vi "initialize averaging variables.vi"(4 "# of  power factor reads to avg":i32, 8 "error in (no error)":errorcluster, 10 "# of ESR reads to  average":i32, 11 "Processing loop variables":T1 {"CurrInverter"."last updated" format="%<%H:%M\n%d/%m/%Y>T"; "CurrInverter"."set flag" items=["False", "True"]}) -> (0 "error out":errorcluster, 3 "Processing loop variables out":T1 {"CurrInverter"."last updated" format="%<%H:%M\n%d/%m/%Y>T"; "CurrInverter"."set flag" items=["False", "True"]})   [LabVIEW 2019, in "Main.lvclass"]
doc: "Developed by Kevin Thompson\nkevin@thompsonengineering.net\n\nCopyright 2020\nThompson Engineering, LLC"
uses:
  Main.lvclass
  DataTypes/Processing loop variables--cluster.ctl
  DataTypes/averaging variables.ctl
  DataTypes/ESR alarm variables.ctl
  Common/DataTypes/Inverter database record v2--cluster.ctl
  Common/DataTypes/inverter info v2--cluster.ctl
  Common/DataTypes/inverter gain range--cluster.ctl
  Common/DataTypes/inverter offset range--cluster.ctl
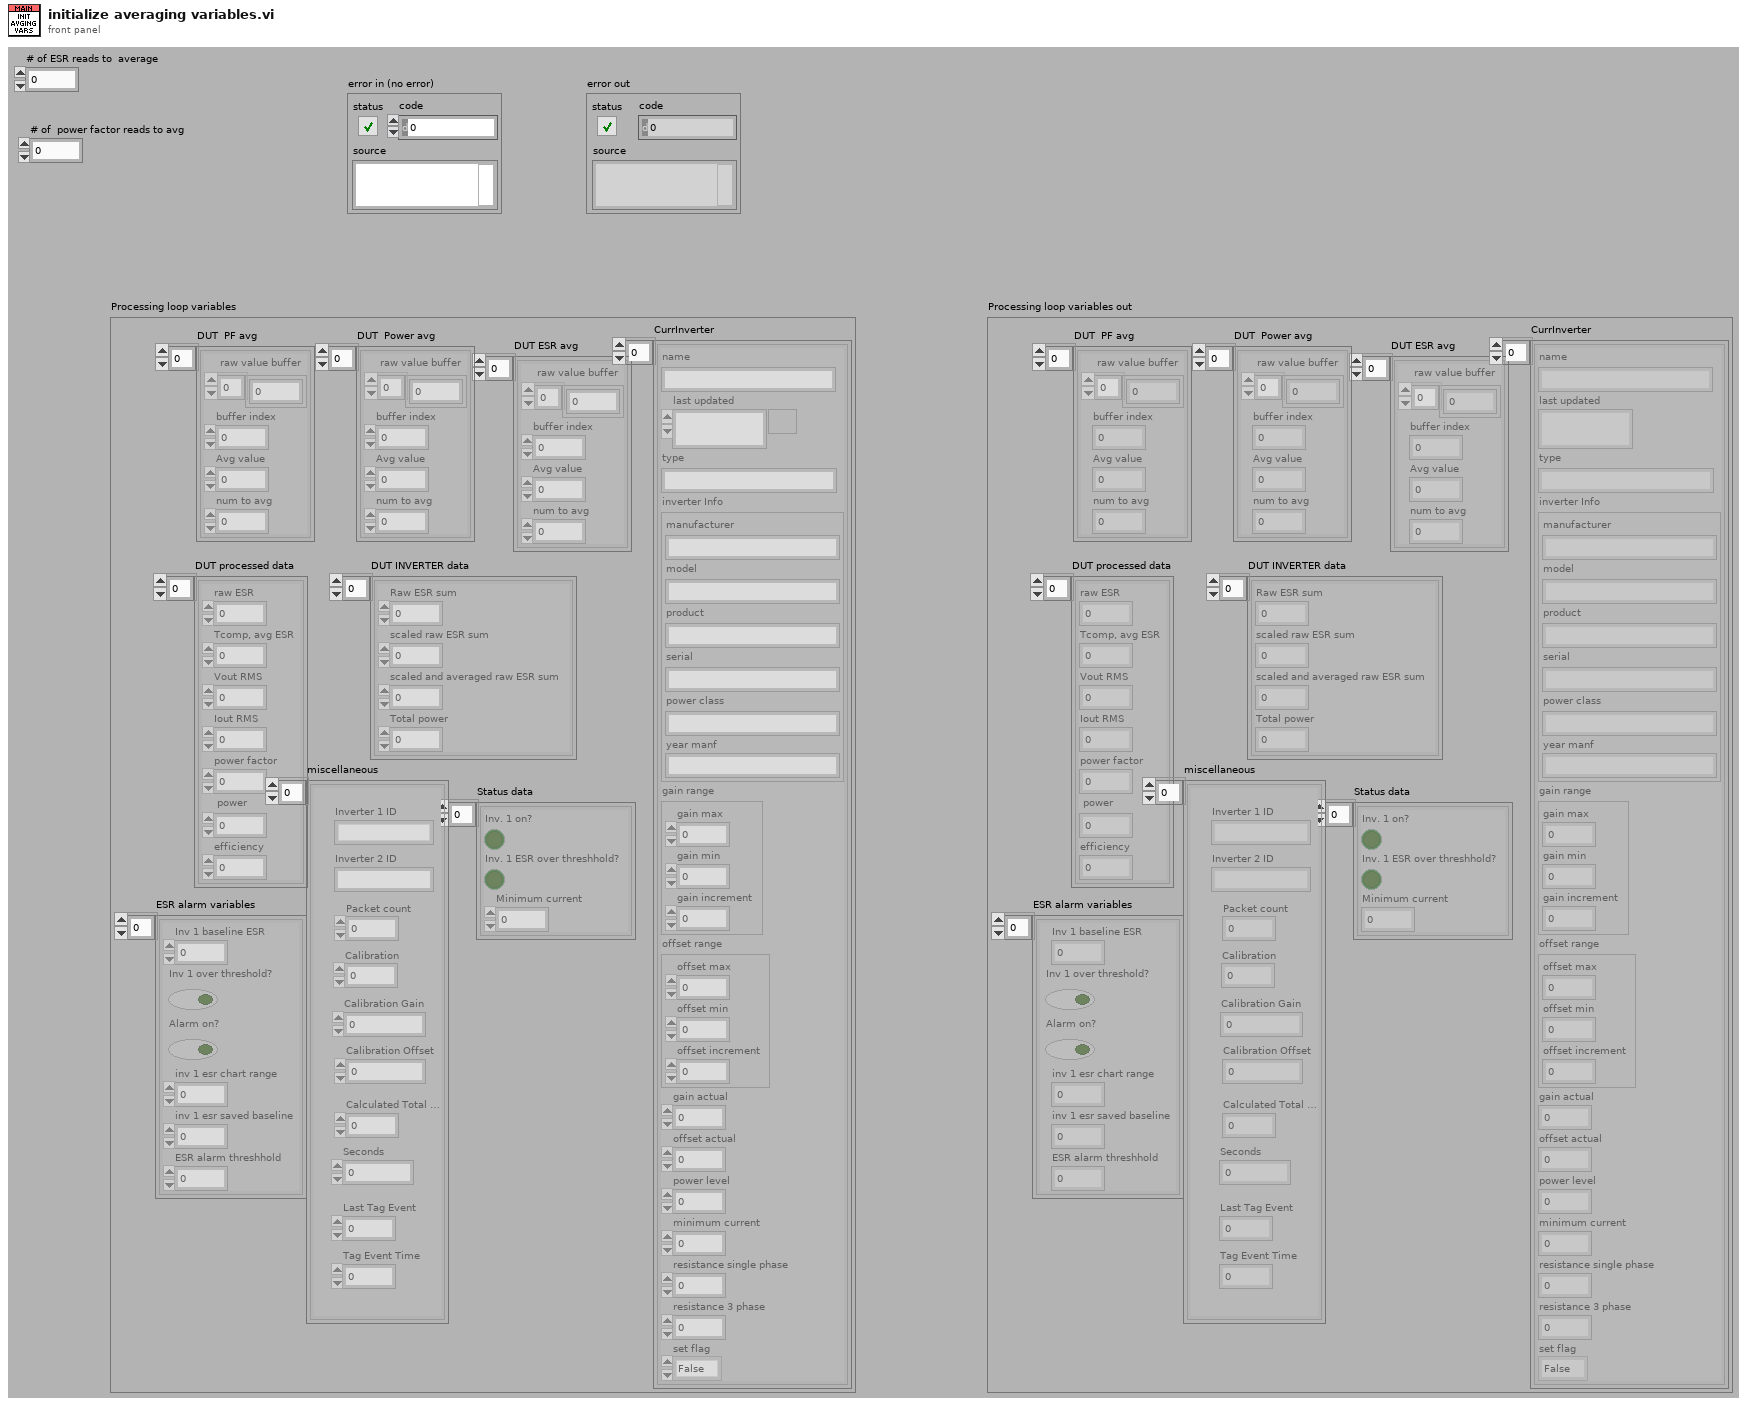
[diagram p1: front panel]
types:
  T1 = typedef "Main.lvclass/Processing loop variables--cluster.ctl" = cluster{"DUT ESR avg":T2[], "DUT  PF avg":T2[], "DUT  Power avg ":T2[], "DUT processed data":cluster{"raw ESR":dbl, "Tcomp, avg ESR":dbl, "Vout RMS":dbl, "Iout RMS":dbl, "power factor":dbl, "power":dbl, "efficiency":dbl}[], "ESR alarm variables":T3[], "Status data":cluster{"Inv. 1 on?":bool, "Inv. 1 ESR over threshhold?":bool, "Minimum current":dbl}[], "CurrInverter":T4[], "miscellaneous":cluster{"Inverter 1 ID":string, "Inverter 2 ID":string, "Packet count":u32, "Calibration":dbl, "Calibration Gain":dbl, "Calibration Offset":dbl, "Calculated Total Power":dbl, "Seconds":dbl, "Last Tag Event":dbl, "Tag Event Time":dbl}[], "DUT INVERTER data":cluster{"Raw ESR sum":dbl, "scaled raw ESR sum":dbl, "scaled and averaged raw ESR sum":dbl, "Total power":dbl}[]}
  T2 = typedef "Main.lvclass/averaging variables.ctl" = cluster{"raw value buffer":dbl[], "buffer index":i32, "Avg value":dbl, "num to avg":i32}
  T3 = typedef "Main.lvclass/ESR alarm variables.ctl" = cluster{"Inv 1 baseline ESR":dbl, "Inv 1 over threshold?":bool, "Alarm on?":bool, "inv 1 esr chart range":dbl, "inv 1 esr saved baseline":dbl, "ESR alarm threshhold":dbl}
  T4 = typedef "Inverter database record v2--cluster.ctl" = cluster{"name":string, "last updated":timestamp, "type":string, "inverter Info":T5, "gain range":T6, "offset range":T7, "gain actual":dbl, "offset actual":dbl, "power level":dbl, "minimum current":dbl, "resistance single phase":dbl, "resistance 3 phase":dbl, "set flag":u16}
  T5 = typedef "inverter info v2--cluster.ctl" = cluster{"manufacturer":string, "model":string, "product":string, "serial":string, "power class":string, "year manf":string}
  T6 = typedef "inverter gain range--cluster.ctl" = cluster{"gain max":dbl, "gain min":dbl, "gain increment":dbl}
  T7 = typedef "inverter offset range--cluster.ctl" = cluster{"offset max":dbl, "offset min":dbl, "offset increment":dbl}
  T8 = cluster{"Raw ESR sum":dbl, "scaled raw ESR sum":dbl, "scaled and averaged raw ESR sum":dbl, "Total power":dbl}
  T9 = cluster{"raw ESR":dbl, "Tcomp, avg ESR":dbl, "Vout RMS":dbl, "Iout RMS":dbl, "power factor":dbl, "power":dbl, "efficiency":dbl}
  T10 = cluster{"raw ESR":dbl, "Tcomp, avg ESR":dbl, "Vout RMS":dbl, "Iout RMS":dbl, "power factor":dbl, "power":dbl, "efficiency":dbl}[]
  T11 = cluster{"Raw ESR sum":dbl, "scaled raw ESR sum":dbl, "scaled and averaged raw ESR sum":dbl, "Total power":dbl}[]
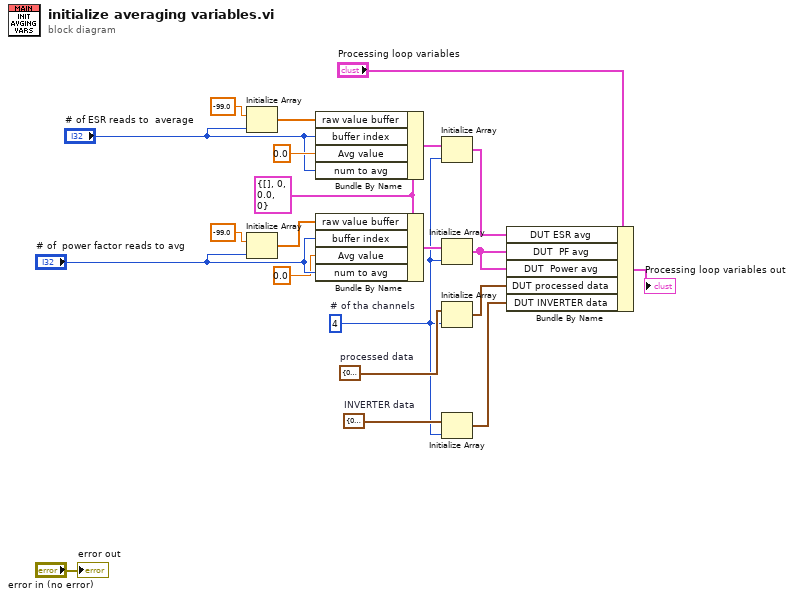
[diagram p0: block diagram]
diagram:
  w3 = T8 {"Raw ESR sum"=0.0, "scaled raw ESR sum"=0.0, "scaled and averaged raw ESR sum"=0.0, "Total power"=0.0}  # INVERTER data
  w7 = T9 {"raw ESR"=0.0, "Tcomp, avg ESR"=0.0, "Vout RMS"=0.0, "Iout RMS"=0.0, "power factor"=0.0, "power"=0.0, "efficiency"=0.0}  # processed data
  w1 = 4  # # of tha channels
  w11 = T2 {"raw value buffer"=[], "buffer index"=0, "Avg value"=0.0, "num to avg"=0} ("Averaging variables")
  n1 = Initialize Array(-99.0 ("element"), "# of ESR reads to  average") -> (w18:dbl[])
  n2 = Initialize Array(-99.0 ("element"), "# of  power factor reads to avg") -> (w15:dbl[])
  n3 = Bundle By Name(cluster=w11, "raw value buffer"=w18, "buffer index"="# of ESR reads to  average", "Avg value"=0.0, "num to avg"="# of ESR reads to  average") -> (w5:T2)
  n4 = Bundle By Name(cluster=w11, "raw value buffer"=w15, "buffer index"="# of  power factor reads to avg", "Avg value"=0.0, "num to avg"="# of  power factor reads to avg") -> (w9:T2)
  n5 = Initialize Array(w5, w1) -> (w4:T2[])
  n6 = Initialize Array(w9, w1) -> (w8:T2[])
  n7 = Initialize Array(w7, w1) -> (w6:T10)
  n8 = Initialize Array(w3, w1) -> (w2:T11)
  n9 = Bundle By Name(cluster="Processing loop variables", "DUT ESR avg"=w4, "DUT  PF avg"=w8, "DUT  Power avg"=w8, "DUT processed data"=w6, "DUT INVERTER data"=w2) -> (→"Processing loop variables out":T1)
  "error out" <- "error in (no error)"
